vi "test_libssh2_channel_close.vi"() -> ()   [LabVIEW 2013, in "libssh2_integration_tests.lvlib"]
uses:
  libssh2_integration_tests.lvlib
  <vilib>/addons/_JKI Toolkits/Caraya/classes/Test/Test.lvclass
  support/support.lvlib
  libssh2/libssh2.lvlib
  <vilib>/addons/_JKI Toolkits/Caraya/classes/Assert/Assert.lvclass
panel:
  out "error out":errorcluster
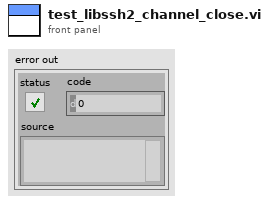
[diagram p1: front panel]
types:
  T1 = typedef "libssh2.lvlib/Session Refnum.ctl" = refnum<k1>
  T2 = typedef "libssh2.lvlib/Channel Refnum.ctl" = refnum<k1>
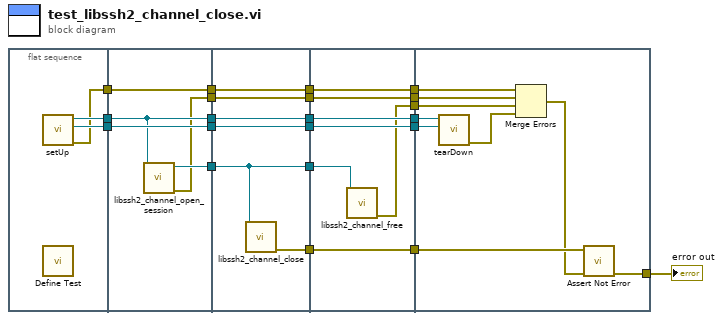
[diagram p0: block diagram]
diagram:
  n1 = flat-sequence {
    tunnel: [w24] -> w21
    tunnel: [w23] -> w20
    tunnel: [w22] -> w7
    tunnel: w21 -> [w28]
    tunnel: w20 -> [w29]
    tunnel: [w28] -> w19
    tunnel: [w29] -> w18
    tunnel: [w27] -> w17
    tunnel: w7 -> [w26]
    tunnel: [w26] -> w6
    tunnel: [w25] -> w2
    tunnel: w19 -> [w35]
    tunnel: w18 -> [w34]
    tunnel: w17 -> [w33]
    tunnel: [w35] -> w16
    tunnel: [w34] -> w15
    tunnel: [w33] -> w14
    tunnel: w6 -> [w32]
    tunnel: [w32] -> w5
    tunnel: [w31] -> w3
    tunnel: w2 -> [w30]
    tunnel: [w30] -> w1
    tunnel: w16 -> [w42]
    tunnel: w15 -> [w41]
    tunnel: w14 -> [w39]
    tunnel: [w42] -> w13
    tunnel: [w41] -> w12
    tunnel: [w40] -> w11
    tunnel: [w38] -> w9
    tunnel: [w37] -> w8
    tunnel: w5 -> [w36]
    tunnel: [w36] -> w4
    tunnel: w3 -> [w40]
    tunnel: w1 -> [w37]
    tunnel: w13 -> [w50]
    tunnel: w12 -> [w49]
    tunnel: w11 -> [w51]
    tunnel: [w48] -> w10
    tunnel: w9 -> [w46]
    tunnel: w8 -> [w45]
    tunnel: w4 -> [w44]
    frame #0 {
      n2 = call "setUp.vi"() -> ("error out"=w22:errorcluster, "connection ID"=w23:refnum<k5>, "session"=w24:T1)  [unwired: 9 in]
      n3 = call <vilib>:"Define Test.vi"() -> ()  [unwired: 10 in, 2 out]
    }
    frame #1 {
      n4 = call "libssh2_channel_open_session.vi"("session"=w28) -> ("error out"=w25:errorcluster, "channel"=w27:T2)  [unwired: 9 in]
    }
    frame #2 {
      n5 = call "libssh2_channel_close.vi"("channel"=w33) -> ("error out"=w31:errorcluster)  [unwired: 10 in]
    }
    frame #3 {
      n6 = call "libssh2_channel_free.vi"("channel"=w39) -> ("error out"=w38:errorcluster)  [unwired: 10 in]
    }
    frame #4 {
      n7 = call "tearDown.vi"("connection ID"=w49, "session"=w50) -> ("error out"=w47:errorcluster)  [unwired: 9 in]
      n8 = Merge Errors(w44, w45, w46, w47) -> (w43:errorcluster)
      n9 = call <vilib>:"Assert Not Error.vi"("error in (no error)"=w43, "Not Error?"=w51) -> ("error out"=w48:errorcluster)  [unwired: 8 in, 1 out]
    }
  }
  "error out" <- w10
